vi "aplicatie II2.vi"() -> ()   [LabVIEW 2011]
panel:
  out "Produs":dbl
  out "Suma":dbl
  out "Numarul 2":dbl
  out "Numarul 1":dbl
  out "Produsul numerelor - reprezentare Meter":dbl(knob)=2400.0 scale=0.0..10000.0
  out "Suma numerelor - reprezentare tip Tank":dbl(slide)=100.0 scale=0.0..200.0
  in  "Numarul 2":u16(slide)=60 scale=0.0..100.0
  in  "Numarul 1":u16(slide)=40 scale=0.0..100.0
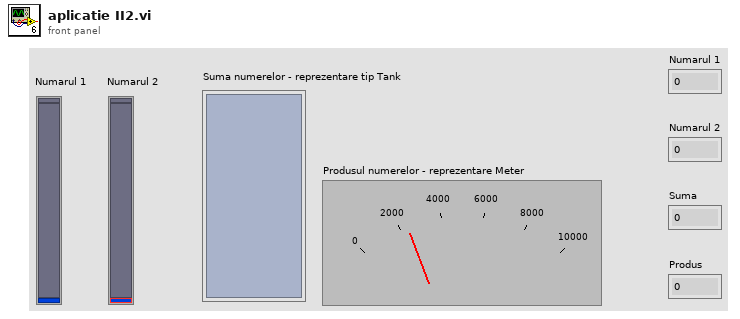
[diagram p1: front panel]
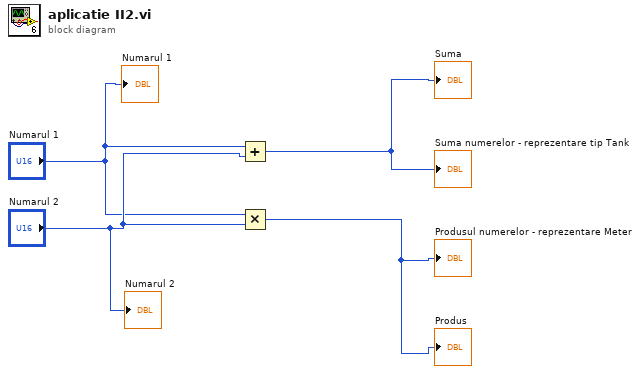
[diagram p0: block diagram]
diagram:
  n1 = Add(x="Numarul 1", y="Numarul 2") -> (x+y=→"Suma numerelor - reprezentare tip Tank" →"Suma":u16)
  n2 = Multiply(x="Numarul 1", y="Numarul 2") -> (x*y=→"Produsul numerelor - reprezentare Meter" →"Produs":u16)
  "Numarul 1" <- "Numarul 1"
  "Numarul 2" <- "Numarul 2"
